vi "add_ExtrapolResults_data.vi"(8 "error in (no error)":errorcluster, 10 "ExtrapolResults":string[](array[string]), 11 "Analysis in":refnum<class "Analysis.lvclass">) -> (0 "error out":errorcluster, 3 "Analysis out":refnum<class "Analysis.lvclass">)   [LabVIEW 2018, in "Analysis.lvclass"]
doc: "adds the Extrapolation Results to the ExtrapolResultsArray\nisoope_name, intercept, RMSE, delta-intercept"
uses:
  Analysis.lvclass
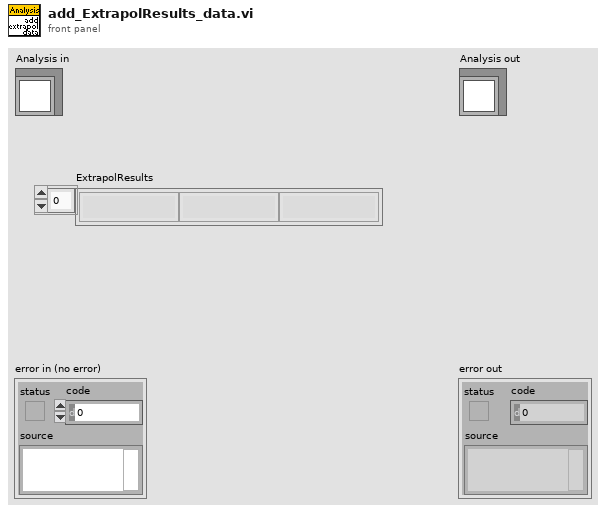
[diagram p1: front panel]
types:
  T1 = typedef "ExtrapolationResultsArray.ctl" = string[][]
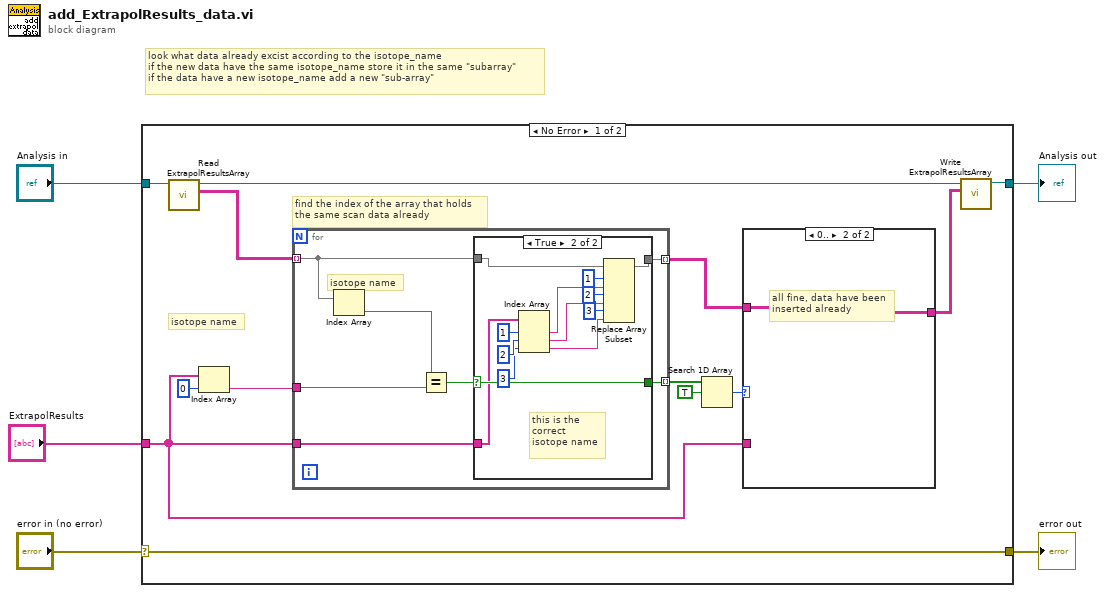
[diagram p0: block diagram]
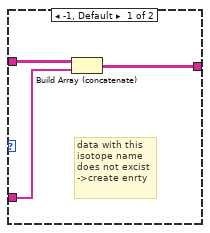
[diagram p2: hidden frame]
diagram:
  # "look what data already excist according to the isotope_name\nif the new data have the same isotope_name store it in the same \"subarray\"\nif the data have a new isotope_name add a new \"sub-array\""
  n1 = case shown="No Error" "error in (no error)" {
    selector: "error in (no error)" -> [w18 w46]
    tunnel: [w18 w46] -> w4
    tunnel: [w15 w45] -> w2
    tunnel: "Analysis in" -> [w17 w45]
    tunnel: "ExtrapolResults" -> [w6 _]
    frame No Error {
      # "find the index of the array that holds\nthe same scan data already"
      # "isotope name"
      n2 = call-dynamic "Read ExtrapolResultsArray.vi"("Analysis in"=w17) -> ("ExtrapolResultsArray"=w13:T1, "Analysis out"=w16:refnum<class "Analysis.lvclass">)  [unwired: 8 in, 1 out]
      n3 = Index Array(array=w6, index=0) -> (element=w11:string)
      n4 = for {
        tunnel: w13 -> [w25] mode=indexing
        tunnel: w11 -> [w29]
        tunnel: [w26] -> w12 mode=indexing
        tunnel: [w24] -> w8 mode=indexing
        tunnel: w6 -> [w28]
        # "isotope name"
        n5 = Index Array(array=w25) -> (element=w23:string)  [unwired: 1 in]
        n6 = Equal?(x=w23, y=w29) -> (x = y?=w27:bool)
        n7 = case shown="True" w27 {
          selector: w27 -> [w31 w44]
          tunnel: w28 -> [_ w40]
          tunnel: [w31 w44] -> w26
          tunnel: w25 -> [w30 w43]
          tunnel: [w30 w42] -> w24
          frame False {
            # "not the right\nsub-array"
          }
          frame True {
            # "this is the\ncorrect\nisotope name"
            n8 = Index Array(array=w40, index #1=1 ("index"), index #2=2 ("index"), index #3=3 ("index")) -> (element #1=w38:string, element #2=w35:string, element #3=w32:string)
            n9 = Replace Array Subset(array=w43, new element #1=w38, index #1=1 ("index"), new element #2=w35, index #2=2 ("index"), new element #3=w32, index #3=3 ("index")) -> (w42:string[])
          }
        }
      }
      n10 = Search 1D Array(1D array=w12, element=TRUE) -> (index of element=w9:i32)  [unwired: 1 in]
      n11 = case shown="0.." w9 {
        tunnel: w8 -> [w20 w22]
        tunnel: w6 -> [w19 _]
        tunnel: [w21 w22] -> w7
        frame -1, Default {
          # "data with this\nisotope name\ndoes not excist\n->create enrty"
          n12 = Build Array (concatenate)(w20, w19) -> (w21:string[][])
        }
        frame 0.. {
          # "all fine, data have been\ninserted already"
        }
      }
      n13 = call-dynamic "Write ExtrapolResultsArray.vi"("ExtrapolResultsArray"=w7, "Analysis in"=w16) -> ("Analysis out"=w15:refnum<class "Analysis.lvclass">)  [unwired: 8 in, 1 out]
    }
    frame Error {
    }
  }
  "error out" <- w4
  "Analysis out" <- w2
